vi "add PID to configuration.vi"(8 "error in":errorcluster, 10 "PID Element in":T1, 11 "Tagbus PID Module configuration in":refnum<class "Tagbus PID Module configuration.lvclass">) -> (0 "error out":errorcluster, 3 "Tagbus PID Module configuration out":refnum<class "Tagbus PID Module configuration.lvclass">)   [LabVIEW 2014, in "Tagbus PID Module configuration.lvclass"]
doc: "This VI takes in a PID Loop configuration, verifies that it's not currently in the Module Configuration object, and adds it to the Module Configuration."
uses:
  Tagbus PID Module configuration.lvclass
  editor node/PID array element.ctl
  Tagbus PID Module configuration.lvclass/Tagbus PID Module configuration.ctl
  PID Loop.lvclass
  editor node/Tagbus PID Module editor node.lvclass
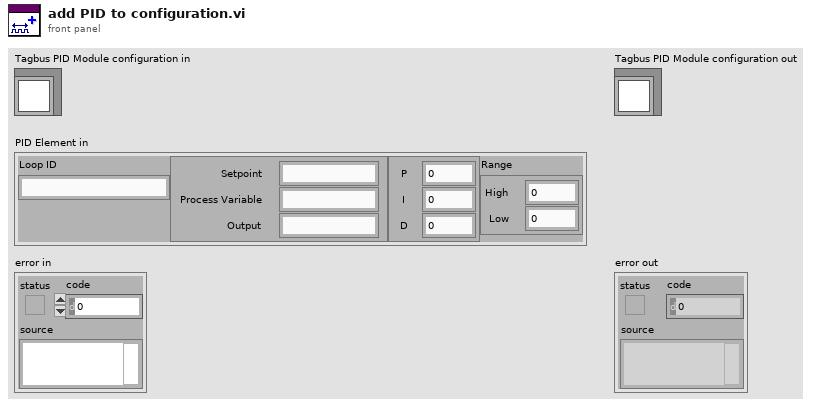
[diagram p1: front panel]
types:
  T1 = typedef "Tagbus PID Module editor node.lvclass/PID array element.ctl" = cluster{"Loop ID":string, "Tags":cluster{"Setpoint":string, "Process Variable":string, "Output":string}, "Gains":cluster{"P":dbl, "I":dbl, "D":dbl}, "Range":cluster{"High":dbl, "Low":dbl}}
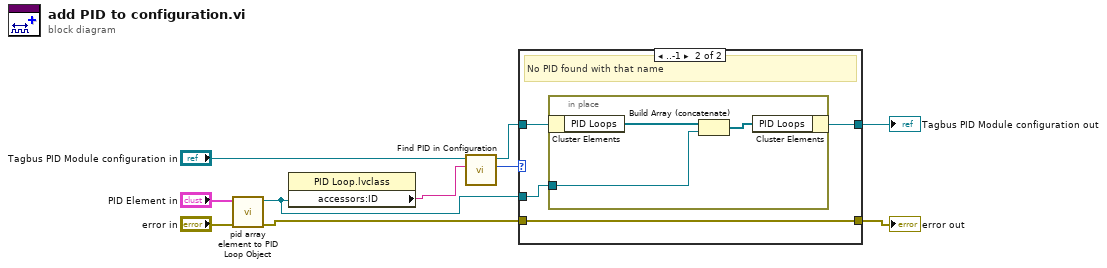
[diagram p0: block diagram]
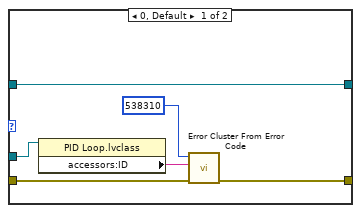
[diagram p2: hidden frame]
diagram:
  n1 = call "pid array element to PID Loop Object.vi"("error in (no error)"="error in", "PID Element in"="PID Element in") -> ("error out"=w6:errorcluster, "PID Loop out"=w1:refnum<class "PID Loop.lvclass">)  [unwired: 8 in]
  n2 = property class="PID Loop.lvclass"(reference=w1) -> ("accessors:ID"=w2:string)  [unwired: 1 in, 2 out]
  n3 = call "Find PID in Configuration.vi"("PID Loop ID in"=w2, "Tagbus PID Module configuration in"="Tagbus PID Module configuration in") -> ("index"=w9:i32, "Tagbus PID Module configuration out"=w8:refnum<class "Tagbus PID Module configuration.lvclass">)  [unwired: 8 in]
  n4 = case shown="..-1" w9 {
    tunnel: w8 -> [w13 w20]
    tunnel: w1 -> [w12 w17]
    tunnel: [w13 w19] -> w7
    tunnel: w6 -> [w15 w18]
    tunnel: [w14 w18] -> w5
    frame 0, Default {
      n5 = property class="PID Loop.lvclass"(reference=w12) -> ("accessors:ID"=w11:string)  [unwired: 1 in, 2 out]
      n6 = call <vilib>:"Error Cluster From Error Code.vi"("error in (no error)"=w15, "error message (\"\")"=w11, "error code (0)"=538310) -> ("error out"=w14:errorcluster)  [unwired: 6 in]
    }
    frame ..-1 {
      # "No PID found with that name"
      n7 = in-place {
        in-place-border: w17 -> [w22]
        n8 = in-place-cluster #1(w20) -> ("PID Loops"=w23:refnum<class "PID Loop.lvclass">[])
        n9 = Build Array (concatenate)(w23, w22) -> (w21:refnum<class "PID Loop.lvclass">[])
        n10 = in-place-cluster #1("PID Loops"=w21) -> (w19:refnum<class "Tagbus PID Module configuration.lvclass">)
      }
    }
  }
  "error out" <- w5
  "Tagbus PID Module configuration out" <- w7
